vi "FlatToRichnixnet_grpc_DbCloseDatabaseRequest.vi"(5 "OutputClusterType":T1, 11 "InputCluster":T3) -> (3 "OutputCluster":T1)   [LabVIEW 2025, in "xnet-grpc_client.lvlib"]
uses:
  nixnet_grpc_DbCloseDatabaseRequest_Flat.ctl
  nidevice_grpc_Session_Flat.ctl
  nixnet_grpc_DbCloseDatabaseRequest.ctl
  nidevice_grpc_Session.ctl
  xnet-grpc_client.lvlib
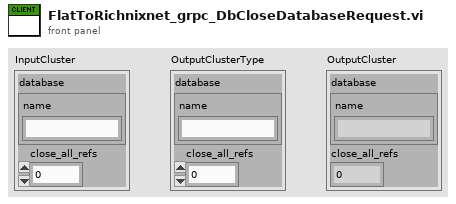
[diagram p1: front panel]
types:
  T1 = typedef "xnet-grpc_client.lvlib/nixnet_grpc_DbCloseDatabaseRequest.ctl" = cluster{"database":T2, "close_all_refs":u32}
  T2 = typedef "xnet-grpc_client.lvlib/nidevice_grpc_Session.ctl" = cluster{"name":string}
  T3 = typedef "xnet-grpc_client.lvlib/nixnet_grpc_DbCloseDatabaseRequest_Flat.ctl" = cluster{"database":T4, "close_all_refs":u32}
  T4 = typedef "xnet-grpc_client.lvlib/nidevice_grpc_Session_Flat.ctl" = cluster{"name":string}
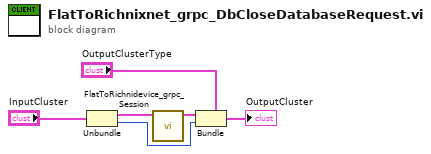
[diagram p0: block diagram]
diagram:
  n1 = Unbundle "Unbundle"("InputCluster") -> ("database"=w3:T4, "close_all_refs"=w1:u32)
  n2 = call "FlatToRichnidevice_grpc_Session.vi"("InputCluster"=w3) -> ("OutputCluster"=w2:T2)  [unwired: 10 in]
  n3 = Bundle "Bundle"(cluster="OutputClusterType", "database"=w2, "close_all_refs"=w1) -> (→"OutputCluster":T1)
